vi "SetRWPermission.vi"(1 "path":path, 5 "error in (no error)":errorcluster) -> (15 "permissions":i16 format="%.0o", 19 "error out":errorcluster)   [LabVIEW 2020, in "SupportLib.lvlib"]
uses:
  SupportLib.lvlib
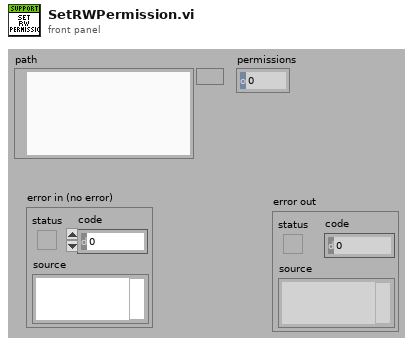
[diagram p1: front panel]
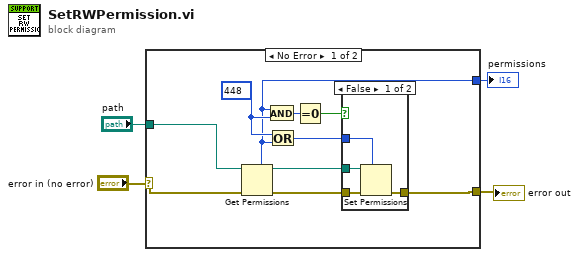
[diagram p0: block diagram]
diagram:
  n1 = case shown="No Error" "error in (no error)" {
    selector: "error in (no error)" -> [w7 w20]
    tunnel: [w6 w20] -> w4
    tunnel: "path" -> [w8 _]
    tunnel: [w5 _] -> w1
    frame No Error {
      w11 = i16 448 ("permissions")
      n2 = Get Permissions(8:w7, 11:w8) -> (0:w9:errorcluster, 3:w12:path, 5:w5:i16)  [unwired: 2 out]
      n3 = And(x=w5, y=w11) -> (x .and. y?=w13:i16)
      n4 = Or(x=w11, y=w5) -> (x .or. y?=w10:i16)
      n5 = Equal To 0?(x=w13) -> (x = 0?=w14:bool)
      n6 = case shown="False" w14 {
        tunnel: w9 -> [w18 w19]
        tunnel: [w17 w19] -> w6
        tunnel: w10 -> [w16 _]
        tunnel: w12 -> [w15 _]
        frame False {
          n7 = Set Permissions(7:w16, 8:w18, 11:w15) -> (0:w17:errorcluster)  [unwired: 2 in, 1 out]
        }
        frame True {
        }
      }
    }
    frame Error {
    }
  }
  "error out" <- w4
  "permissions" <- w1
